vi "PCO_Save.vi"(8 "entrée d'erreur (pas d'erreur)":errorcluster, 9 "raw_image_list (U16)":u16[][][](array[numeric]), 10 "meta_data_list":T1(array[cluster]), 11 "SavePath":path) -> (0 "sortie d'erreur":errorcluster)   [LabVIEW 2026]
uses:
  <vilib>/Utility/file.llb/Write Delimited Spreadsheet (string).vi
  <instrlib>/PCO_SDK/File Group 0/vi.lib/Excelitas PCO GmbH/pco.labview/pco.recorder/Recorder.lvlib
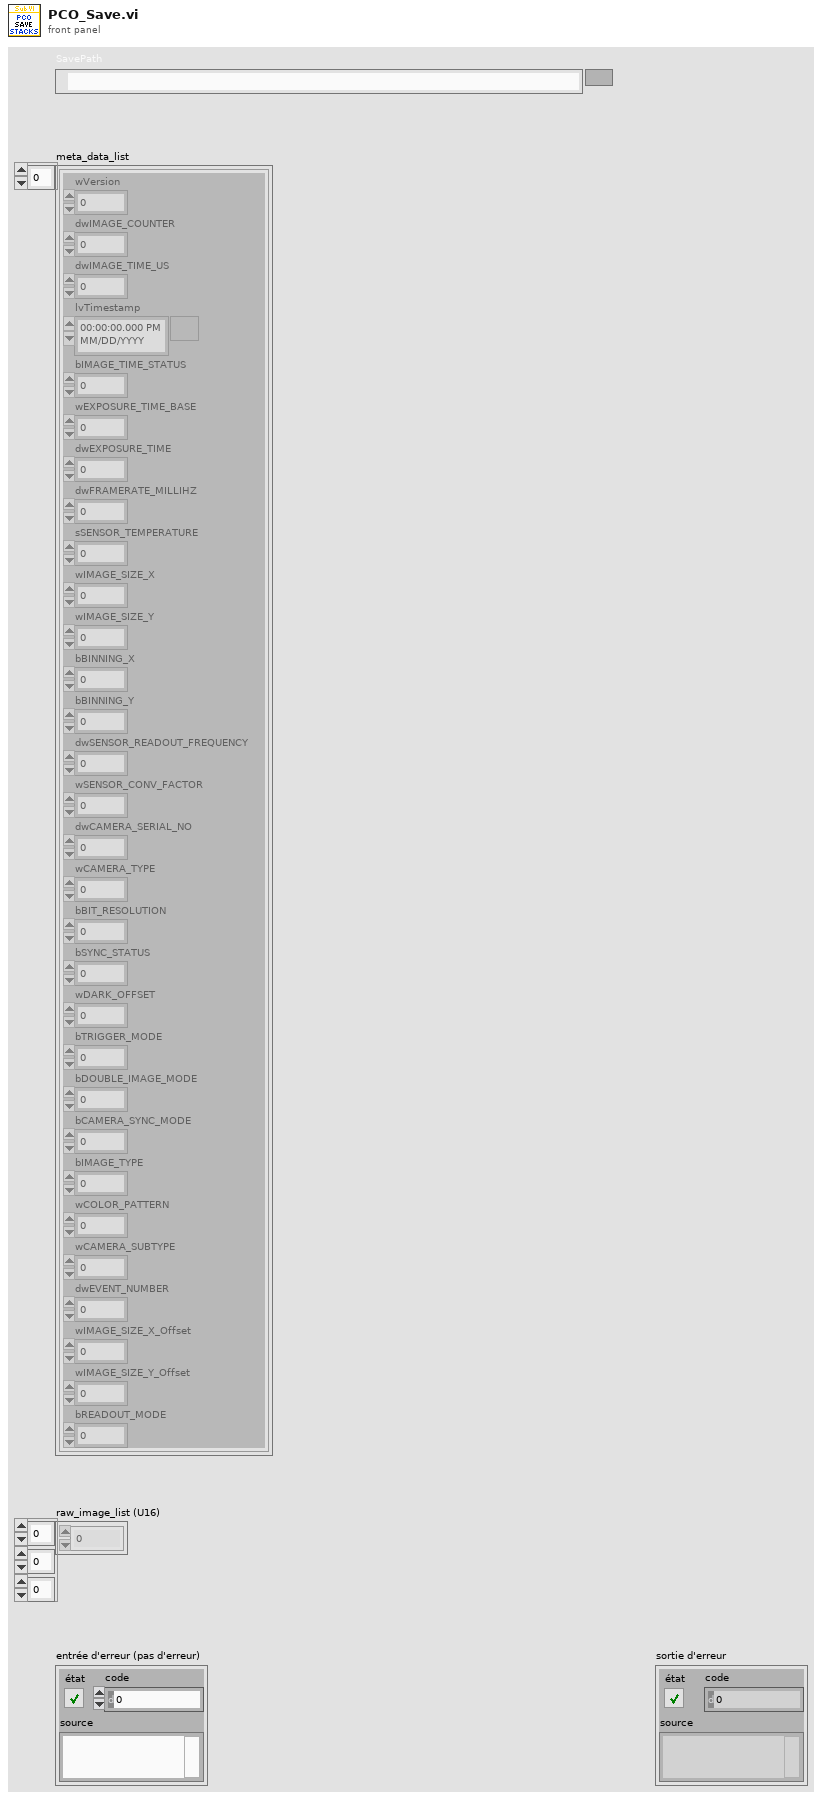
[diagram p1: front panel]
types:
  T1 = cluster{"wVersion":u16, "dwIMAGE_COUNTER":u32, "dwIMAGE_TIME_US":u32, "lvTimestamp":timestamp, "bIMAGE_TIME_STATUS":u8, "wEXPOSURE_TIME_BASE":u16, "dwEXPOSURE_TIME":u32, "dwFRAMERATE_MILLIHZ":u32, "sSENSOR_TEMPERATURE":i16, "wIMAGE_SIZE_X":u16, "wIMAGE_SIZE_Y":u16, "bBINNING_X":u8, "bBINNING_Y":u8, "dwSENSOR_READOUT_FREQUENCY":u32, "wSENSOR_CONV_FACTOR":u16, "dwCAMERA_SERIAL_NO":u32, "wCAMERA_TYPE":u16, "bBIT_RESOLUTION":u8, "bSYNC_STATUS":u8, "wDARK_OFFSET":u16, "bTRIGGER_MODE":u8, "bDOUBLE_IMAGE_MODE":u8, "bCAMERA_SYNC_MODE":u8, "bIMAGE_TYPE":u8, "wCOLOR_PATTERN":u16, "wCAMERA_SUBTYPE":u16, "dwEVENT_NUMBER":u32, "wIMAGE_SIZE_X_Offset":u16, "wIMAGE_SIZE_Y_Offset":u16, "bREADOUT_MODE":u8}[]
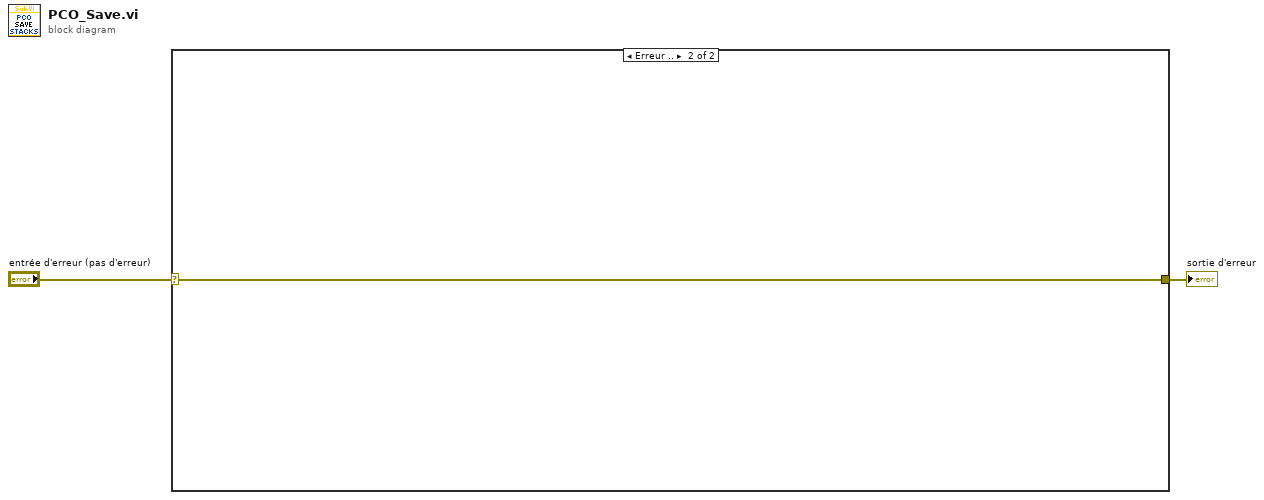
[diagram p0: block diagram]
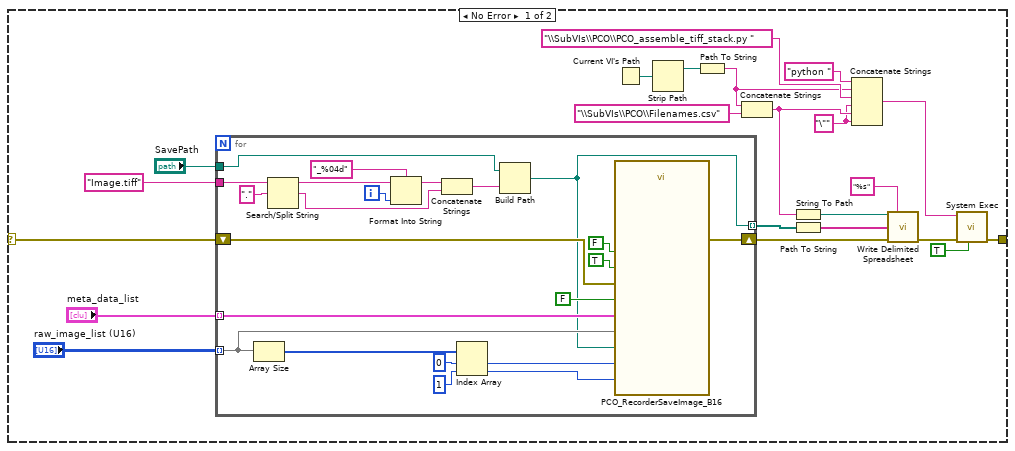
[diagram p2: hidden frame]
diagram:
  n1 = case shown="Erreur .." "entrée d'erreur (pas d'erreur)" {
    selector: "entrée d'erreur (pas d'erreur)" -> [w3 w47]
    tunnel: [w4 w47] -> w2
    frame No Error {
      w12 = "\"" ("chaîne")
      n2 = for {
        tunnel: "raw_image_list (U16)" -> [w46] mode=indexing
        tunnel: "Image.tiff" -> [w38]
        tunnel: "SavePath" -> [w37]
        shift-right: [w35] -> w9
        shift-left: w3 -> [w36]
        tunnel: "meta_data_list" -> [w34] mode=indexing
        tunnel: [w25] -> w20 mode=indexing
        i -> [w39]
        n3 = Array Size(array=w46) -> (size(s)=w30:i32[])
        n4 = Search/Split String(string=w38, search string/char (-)=".") -> (substring before match=w43:string, match + rest of string=w44:string)  [unwired: 1 in, 1 out]
        n5 = Format Into String(format string="_%04d", initial string=w43, w39) -> (resulting string=w45:string)  [unwired: 1 in, 1 out]
        n6 = Concatenate Strings(w45, w44) -> (w40:string)
        n7 = Index Array(array=w30, index #1=0 ("index"), index #2=1 ("index")) -> (element #1=w28:i32, element #2=w27:i32)
        n8 = Build Path(base path=w37, name or relative path=w40) -> (appended path=w25:path)
        n9 = call <instrlib>:"PCO_RecorderSaveImage_B16.vi"("pImgBuf"=w46, "wWidth"=w27, "wHeight"=w28, "szFilePath"=w25, "error in (no error)"=w36, "isColor"=FALSE, "bIsBitmap"=FALSE, "PCO_METADATA_STRUCT"=w34, "bOverwrite"=TRUE) -> ("error out"=w35:errorcluster)  [unwired: 9 in, 1 out]
      }
      n10 = Current VI's Path() -> (path=w8:path)
      n11 = Strip Path(path=w8) -> (stripped path=w7:path)  [unwired: 1 out]
      n12 = Path To String(path=w7) -> (string=w15:string)
      n13 = Concatenate Strings(w15, "\\SubVIs\\PCO\\Filenames.csv" ("chaîne")) -> (w13:string)
      n14 = String To Path(string=w13) -> (path=w17:path)
      n15 = Path To String(path=w20) -> (string=w19:string[])
      n16 = Concatenate Strings("python " ("chaîne"), w15, "\\SubVIs\\PCO\\PCO_assemble_tiff_stack.py " ("chaîne"), w12, w13, w12) -> (w11:string)
      n17 = call-poly <vilib>:"Write Delimited Spreadsheet.vi"("file path (dialog if empty)"=w17, "format (%s)"="%s" ("format (%.3f)"), "1D data"=w19, "error in (no error)"=w9) -> ("error out"=w10:errorcluster)  [unwired: 10 in, 1 out]
      n18 = call <vilib>:"System Exec.vi"("run minimized? (F)"=TRUE, "error in (no error)"=w10, "command line"=w11) -> ("error out"=w4:errorcluster)  [unwired: 5 in, 3 out]
    }
    frame Error {
    }
  }
  "sortie d'erreur" <- w2
